vi "Get TableParts.vi"(8 "error in":errorcluster, 10 "Sheet Name":string, 11 "SpreadsheetDoc in":refnum<k24>) -> (0 "error out":errorcluster, 1 "SheetName":string, 2 "TableParts":refnum<k24>, 3 "SpreadsheetDoc out":refnum<k24>)   [LabVIEW 2019, in "Open Xml.lvlib"]
uses:
  Open Xml.lvlib
  D:/git/Open-Xml-LabVIEW/Source/DocumentFormat.OpenXml.dll
  DocumentFormat.OpenXml.dll
  D:/git/Open-Xml-LabVIEW/Source/DocumentFormat.OpenXml.Framework.dll
  DocumentFormat.OpenXml.Framework.dll
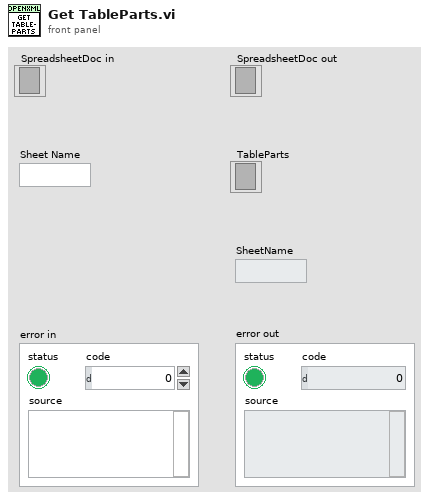
[diagram p1: front panel]
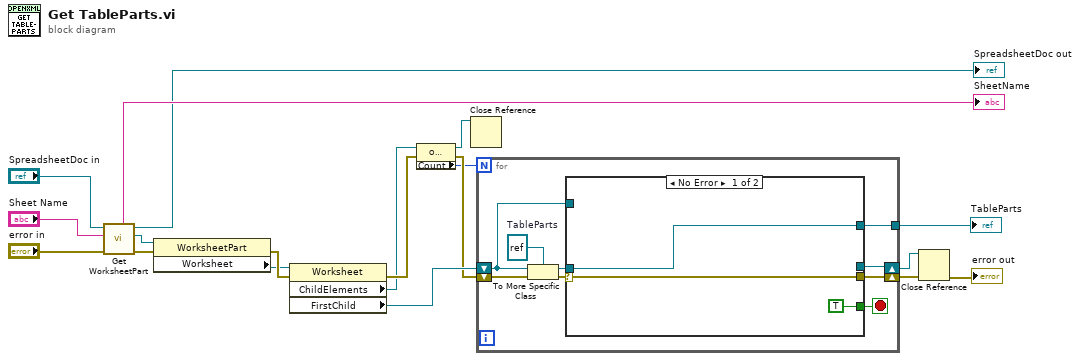
[diagram p0: block diagram]
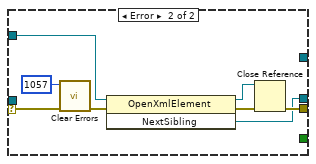
[diagram p2: hidden frame]
diagram:
  n1 = call "Get WorksheetPart.vi"("error in"="error in", "Sheet Name"="Sheet Name", "SpreadsheetDoc in"="SpreadsheetDoc in") -> ("error out"=w7:errorcluster, "WorksheetPart"=w8:refnum<k24>, "SpreadsheetDoc out"=→"SpreadsheetDoc out":refnum<k24>, "SheetName"=→"SheetName":string)  [unwired: 5 in]
  n2 = property class="WorksheetPart"(reference=w8, error in=w7) -> (error out=w10:errorcluster, "Worksheet"=w9:refnum<k24>)  [unwired: 1 out]
  n3 = property class="Worksheet"(reference=w9, error in=w10) -> (error out=w14:errorcluster, "ChildElements"=w11:refnum<k24>, "FirstChild"=w16:refnum<k24>)  [unwired: 1 out]
  n4 = property class="OpenXmlElementList"(reference=w11, error in=w14) -> (reference out=w13:refnum<k24>, error out=w15:errorcluster, "Count"=w12:i32)
  n5 = Close Reference(reference=w13) -> ()  [unwired: 1 in, 1 out]
  n6 = for {
    N: w12 -> [_]
    shift-right: [w25] -> w17
    shift-left: w15 -> [w28]
    shift-right: [w23] -> w18
    shift-left: w16 -> [w24]
    tunnel: [w20] -> w19
    stop <- w22 stop-if-true
    w27 = refnum<k24> refnum  # TableParts
    n7 = To More Specific Class(target class=w27, reference=w24, error in=w28) -> (specific class reference=w21:refnum<k24>, error out=w26:errorcluster)
    n8 = case shown="No Error" w26 {
      selector: w26 -> [w31 w39]
      tunnel: [w31 w34] -> w25
      tunnel: w24 -> [_ w35]
      tunnel: [_ w32] -> w23
      tunnel: [TRUE _] -> w22
      tunnel: w21 -> [w29 _]
      tunnel: [w29 _] -> w20
      frame No Error {
      }
      frame Error {
        n9 = call <vilib>:"Clear Errors.vi"("error in (no error)"=w39, "specific error code to clear (0: all)"=1057) -> ("error out"=w38:errorcluster)  [unwired: 4 in, 1 out]
        n10 = invoke class="OpenXmlElement" method="NextSibling"(reference=w35, error in=w38) -> (reference out=w33:refnum<k24>, error out=w36:errorcluster, "NextSibling"=w32:refnum<k24>)  [unwired: 1 in]
        n11 = Close Reference(reference=w33, error in (no error)=w36) -> (error out=w34:errorcluster)
      }
    }
  }
  "TableParts" <- w19
  n12 = Close Reference(reference=w18, error in (no error)=w17) -> (error out=→"error out":errorcluster)
